vi "Express VI Framework Strings Global.vi"() -> ()   [LabVIEW 2021]
panel:
  in  "Unsupported Channel":string="Unsupported channel"
  in  "Status Message.Invalid Data.Invalid Timer IRQ Config":string="        Invalid configuration. Check the callback VI path."
  in  "Status Message.Invalid Data.Invalid IRQ Config":string="        Invalid configuration. Check the channel or the callback VI path."
  in  "Status Message.Invalid Data.Invalid Sample Rate":string="        Invalid sample rate. Click the Validate button to coerce to the nearest valid sample rate."
  in  "Status Message.Invalid Data.Invalid Frequency":string="        Invalid frequency. Click the Validate button to coerce to the nearest valid frequency."
  in  "CS Lines String":string="You can use the chip select (CS) lines on the SPI port as DIO lines. The CS lines have 40 kOhm pullup resistors to 3.3 V."
  in  "A/UART String":string="The UART receive input line (RX) and transmit output line (TX) are electrically identical to DIO lines 0 to 13 on the MXP connectors. Like the DIO lines, the UART lines have 40 kOhm pullup resistors to 3.3 V."
  in  "Status Message.Invalid Data.Invalid Target":string="        The current target does not support the channel."
  in  "Status Message.Invalid Data.Uncheck All":string="        Select at least one channel."
  in  "Status Message.Invalid Data.LED Target Change":string="        The current target does not support the previously configured LED channels."
  in  "Status Message.Invalid Data.Illegal Alias":string="        The custom channel name contains invalid characters."
  in  "Warning Pane.Target Error Message":string="The target does not support this Express VI. Click the Help button to get the information about the targets that support this Express VI."
  in  "PWM/RELAY String":string="Voltage levels on DIO lines:\n- MXP, DIO, I2C, and SPI ports: 3.3 V\n- PWM and Relay ports: 5 V"
  in  "RS-232 String":string="The RS-232 receive input line and transmit output line are compliant with TIA/EIA-232-F voltage levels. The following are the valid voltage levels:\n- Logic one voltage level ranges from -5 V to -15 V.\n- Logic zero voltage level ranges from +5 V to +15 V."
  in  "DIO Lines String":string="When a DIO line is floating, it floats in the direction of the pull resistor. A DIO line may be floating when the %s is starting up or powering down, or when the DIO line is configured as an input. \n\nYou can add a stronger resistor to a DIO line to make it float in the opposition direction."
  in  "Warning Pane.Notice Message":string="To switch between personalities, you also can right-click the current target in the Project Explorer window."
  in  "Warning Pane.Warning Message":string="Changing the FPGA personality impacts all the VIs under the current target."
  in  "Warning Pane.Error Message":string="This Express VI is not supported in the %s FPGA personality because the personality does not support the functionality or channel."
  in  "Status Message.No Connector":string="No connector is needed."
  in  "Status Message.Invalid Data":string="        The current FPGA personality or target does not support the channel."
  in  "Disclaimer.In Dialog":string="This window shows the underlying code of the Express VI."
  in  "Show Preview.On State":string="<< Configuration"
  in  "Show Preview.Off State":string="View Code"
  in  "Status Message.Preview":string="Generating Code..."
  in  "Status Message.Scripting":string="Scripting Block Diagram..."
  in  "Status Message.Loading":string="Loading Dialog..."
  in  "Status Message.Update":string="Updating..."
  # "This global maintains strings displayed in the Express vi Framework (Express VI Config Dialog.vi)\n-- Name Format: <Control Name>.<Action>\n-- To modify a string, edit its contents and set Data Operations >>Make Current Value Default"
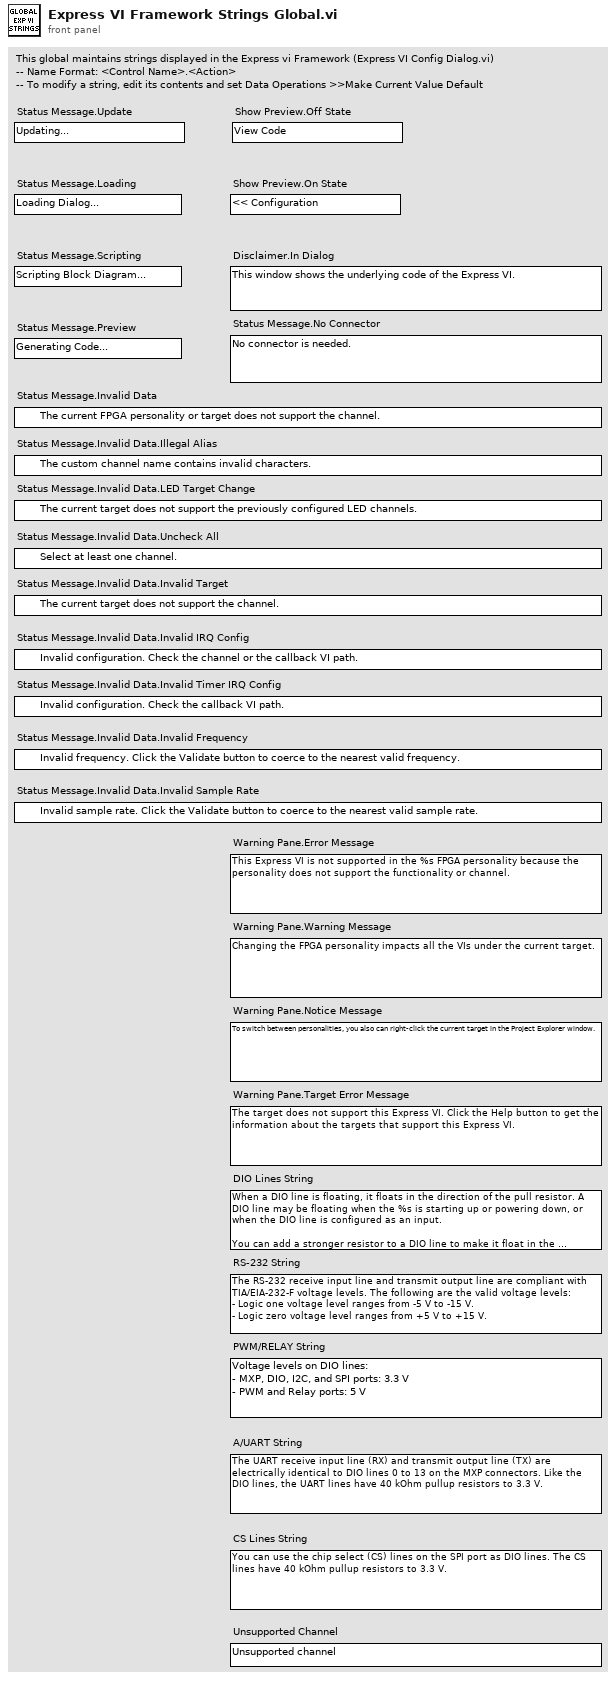
[diagram p1: front panel]
diagram:
